vi "PPMS PS Client watch dog.vi"() -> ()   [LabVIEW 2025]
panel:
  out "Error log":string
  out "LHe level":dbl format="%#_4g"
  # "Run this VI in parallel with the PS Control.VI for PPMS.\n\nIf a network error is detected (appear as zero LHe level), this VI\nresets the PS Control.VI to re-establish the network connection."
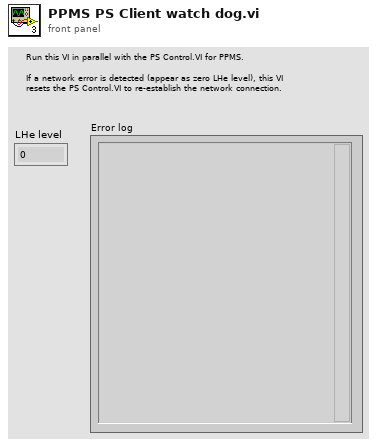
[diagram p1: front panel]
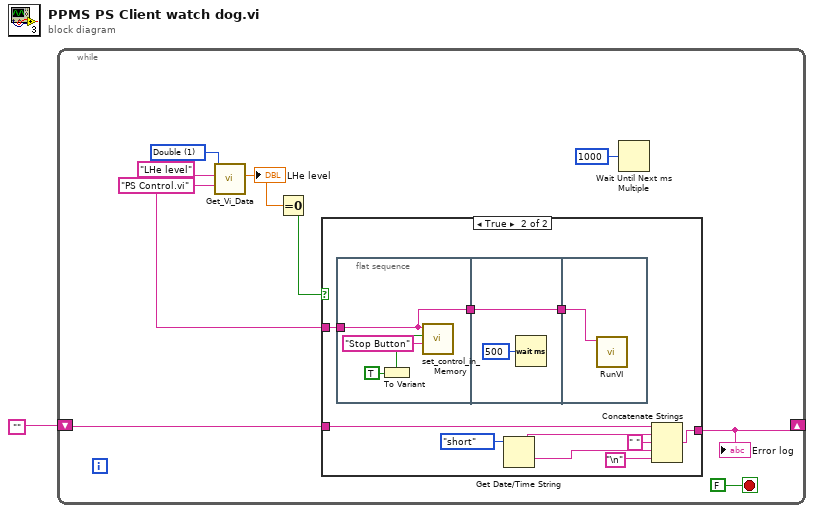
[diagram p0: block diagram]
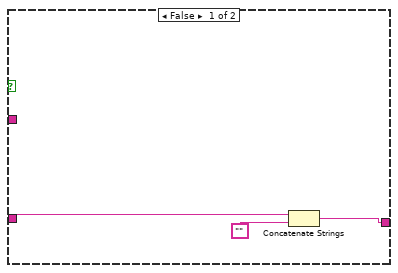
[diagram p2: hidden frame]
diagram:
  n1 = while {
    shift-right: [w3] -> _
    shift-left: "" -> [w4]
    stop <- FALSE stop-if-true
    w9 = u16 1 items=["String", "Double", "Boolean", "Variant"] ("Data Type")
    w7 = "PS Control.vi" ("VI name")
    n2 = call "Get_Vi_Data.vi"("Data Type"=w9, "VI name"=w7, "Control Name"="LHe level") -> ("Data (Double)"=w8:dbl)  [unwired: 4 in, 4 out]
    "LHe level" <- w8
    n3 = Equal To 0?(x=w8) -> (x = 0?=w2:bool)
    n4 = case shown="True" w2 {
      tunnel: w7 -> [_ w23]
      tunnel: w4 -> [w13 w20]
      tunnel: [w11 w19] -> w3
      frame False {
        n5 = Concatenate Strings(w13, "") -> (w11:string)
      }
      frame True {
        n6 = flat-sequence {
          tunnel: w23 -> [w24]
          tunnel: [w24] -> w22
          tunnel: w22 -> [w27]
          tunnel: [w27] -> w21
          tunnel: w21 -> [w29]
          frame #0 {
            w25 = TRUE
            n7 = To Variant(anything=w25) -> ()  [unwired: 1 out]
            n8 = call "set_control_in_Memory.vi"("Control Name"="Stop Button", "Value"=w25, "VI Name"=w24) -> ()  [unwired: 2 in, 1 out]
          }
          frame #1 {
            n9 = Wait (ms)(milliseconds to wait=u32 500) -> ()  [unwired: 1 out]
          }
          frame #2 {
            n10 = call "RunVI.vi"("String"=w29) -> ()  [unwired: 10 in, 1 out]
          }
        }
        n11 = Get Date/Time String(date format (0)=enum16{"short", "long", "abbreviated"}."short") -> (date string=w18:string, time string=w15:string)  [unwired: 2 in]
        n12 = Concatenate Strings(w20, w18, " " ("string"), w15, "\n") -> (w19:string)
      }
    }
    "Error log" <- w3
    n13 = Wait Until Next ms Multiple(millisecond multiple=u32 1000) -> ()  [unwired: 1 out]
  }
